vi "getExtProcFolderPath.vi"(8 "error in (no error)":errorcluster) -> (0 "error out":errorcluster, 3 "ApplicationPath":path)   [LabVIEW 2011]
uses:
  050 - CONFIG/00 - ApplicationConfig/Ctrls/EnumFgvConfigCommand.ctl
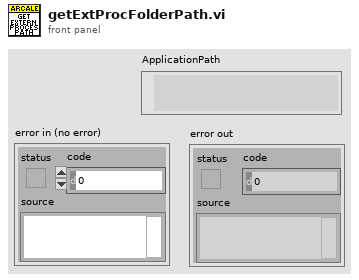
[diagram p1: front panel]
types:
  T1 = typedef "EnumFgvConfigCommand.ctl" = enum16{"Load", "Get", "Set", "Save To Disk"}
  T2 = enum32{"invalid app kind", "Development System", "Run Time System", "Student Edition", "Embedded LabVIEW", "Evaluation", "Custom"}
  T3 = typedef "BenchConfig.ctl" = cluster{"Cfg":string}
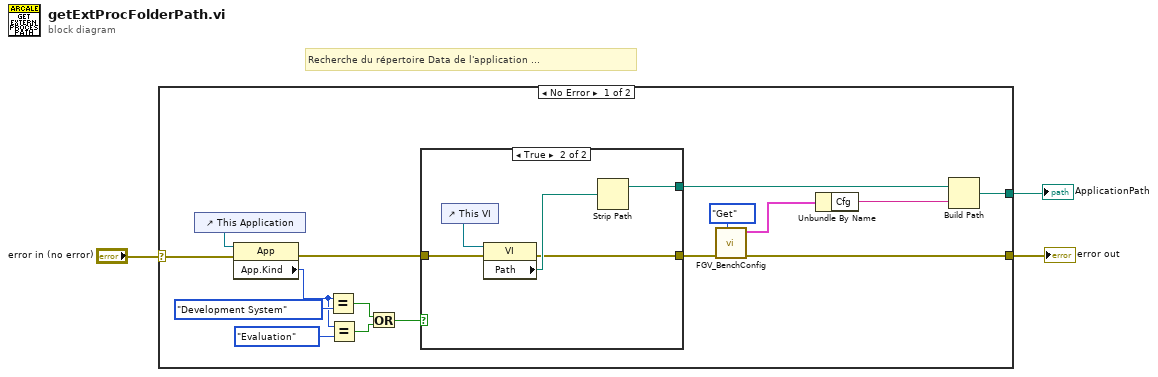
[diagram p0: block diagram]
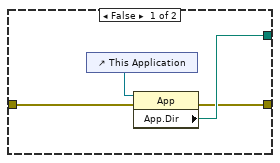
[diagram p2: hidden frame]
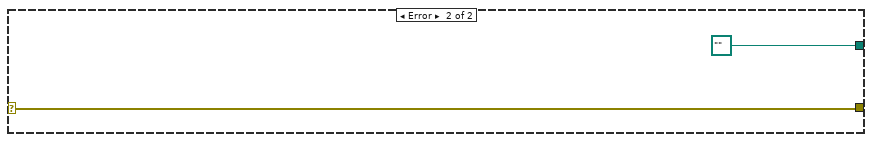
[diagram p3: hidden frame]
diagram:
  # "Recherche du répertoire Data de l'application ..."
  n1 = case shown="No Error" "error in (no error)" {
    selector: "error in (no error)" -> [w16 w29]
    tunnel: [w7 path "" ("appended path")] -> w3
    tunnel: [w4 w29] -> w1
    frame No Error {
      n2 = control-ref of="This Application"() -> (w19:refnum<vi>)
      n3 = property class="App"(reference=w19, error in=w16) -> (error out=w17:errorcluster, "App.Kind"=w15:T2)  [unwired: 1 out]
      n4 = Equal?(x=w15, y=T2."Development System") -> (x = y?=w12:bool)
      n5 = Equal?(x=w15, y=T2."Evaluation") -> (x = y?=w13:bool)
      n6 = Or(x=w12, y=w13) -> (x .or. y?=w11:bool)
      n7 = case shown="True" w11 {
        tunnel: [w22 w26] -> w8
        tunnel: w17 -> [w21 w25]
        tunnel: [w20 w24] -> w5
        frame False {
          n8 = control-ref of="This Application"() -> (w23:refnum<vi>)
          n9 = property class="App"(reference=w23, error in=w21) -> (error out=w20:errorcluster, "App.Dir"=w22:path)  [unwired: 1 out]
        }
        frame True {
          n10 = control-ref of="This VI"() -> (w27:refnum<vi>)
          n11 = property class="VI"(reference=w27, error in=w25) -> (error out=w24:errorcluster, "Path"=w28:path)  [unwired: 1 out]
          n12 = Strip Path(path=w28) -> (stripped path=w26:path)  [unwired: 1 out]
        }
      }
      n13 = call "FGV_BenchConfig.vi"("Command"=EnumFgvConfigCommand."Get", "error in (no error)"=w5) -> ("error out"=w4:errorcluster, "BenchConfigOut"=w9:T3)  [unwired: 8 in]
      n14 = Unbundle By Name(w9) -> ("Cfg"=w6:string)
      n15 = Build Path(base path=w8, name or relative path=w6) -> (appended path=w7:path)
    }
    frame Error {
    }
  }
  "error out" <- w1
  "ApplicationPath" <- w3
